vi "Send Configure TV Trigger Source [TV].vi"(5 "tv trigger polarity (Positive)":i32(ring)=1 items=["Positive"=1, "Negative"=2], 6 "tv event (Field 1)":i32(ring)=1 items=["Field 1"=1, "Field 2"=2, "Any Field"=3, "Any Line"=4, "Line Number"=5], 7 "Message Priority (Normal)":T1=enum."Normal", 8 "error in (no error)":errorcluster, 9 "tv signal format (NTSC)":i32(ring)=1 items=["NTSC"=1, "PAL"=2, "SECAM"=3], 10 "trigger source (\"CHANNEL1\")":string(combo)="CHANNEL1", 11 "Message Enqueuer":refnum<class "Message Enqueuer.lvclass">) -> (0 "error out":errorcluster, 3 "Message Enqueuer out":refnum<class "Message Enqueuer.lvclass">)   [LabVIEW 2013, in "CS++Scope.lvlib" / "Configure TV Trigger Source [TV] Msg.lvclass"]
doc: "This VI sends the message to an actor."
uses:
  Configure TV Trigger Source [TV] Msg.lvclass
  <vilib>/ActorFramework/Message Enqueuer/Message Enqueuer.lvclass
  <vilib>/ActorFramework/Message Enqueuer/Message Priority.ctl
  Configure TV Trigger Source [TV] Msg.lvclass/Configure TV Trigger Source [TV] Msg.ctl
  <vilib>/ActorFramework/Message Enqueuer/Message Enqueuer.lvclass/Message Enqueuer.ctl
  <vilib>/ActorFramework/Message Priority Queue/Priority Enqueue.vi
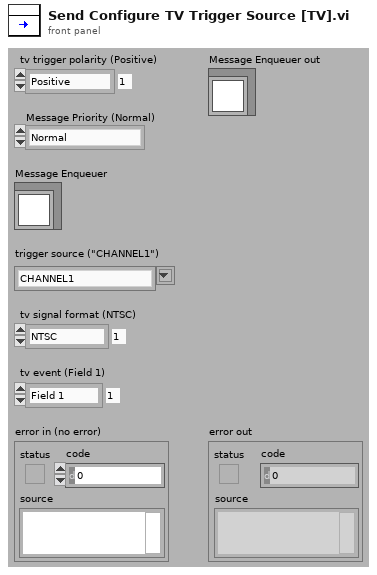
[diagram p1: front panel]
types:
  T1 = typedef "Actor Framework.lvlib/Message Enqueuer.lvclass/Message Priority.ctl" = enum16{"Low", "Normal", "High"}
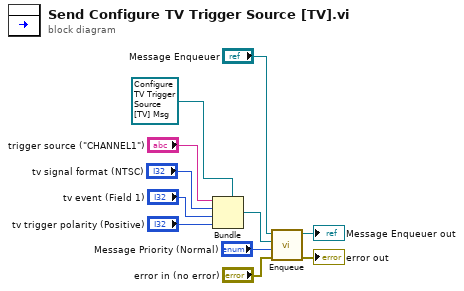
[diagram p0: block diagram]
diagram:
  n1 = Bundle(cluster=refnum<class "Configure TV Trigger Source [TV] Msg.lvclass"> refnum ("Object"), "trigger source (\"CHANNEL1\")", "tv signal format (NTSC)", "tv event (Field 1)", "tv trigger polarity (Positive)") -> (w7:refnum<class "Configure TV Trigger Source [TV] Msg.lvclass">)
  n2 = call <vilib>:"Enqueue.vi"("error in (no error)"="error in (no error)", "Message Priority (Normal)"="Message Priority (Normal)", "Message"=w7, "Message Enqueuer in"="Message Enqueuer") -> ("error out"=→"error out":errorcluster, "Message Enqueuer out"=→"Message Enqueuer out":refnum<class "Message Enqueuer.lvclass">)  [unwired: 6 in]
